vi "Kaelus PFE Initialize.vi"(8 "error in (no error)":errorcluster, 11 "Configuration":T2={"BusType"=enum."USB", "Card"=0, "USB"="", "IP"=0, "COM"=1, "Baud Rate"=enum."9600"}) -> (0 "error out":errorcluster {"code" format="%.0x"}, 3 "DAQmx Dev Name (FEModule)":string, 5 "Kaelus PFE":T1)   [LabVIEW 2011]
uses:
  TypeDefs/Kaelus PFE Configuration.ctl
  TypeDefs/Kaelus PFE Instrument Info.ctl
  OpenG.LIB/file/file.llb/File Exists - Scalar__ogtk.vi
  <vilib>/Utility/config.llb/Read Key (String).vi
  <vilib>/Utility/config.llb/NI_LVConfig.lvlib
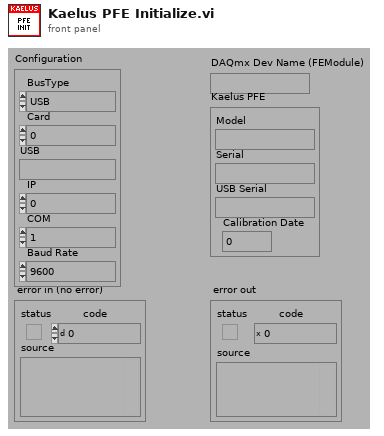
[diagram p1: front panel]
types:
  T1 = typedef "Kaelus PFE Instrument Info.ctl" = cluster{"Model":string, "Serial":string, "USB Serial":string, "Calibration Date":dbl}
  T2 = typedef "Kaelus PFE Configuration.ctl" = cluster{"BusType":enum32{"PCI/ISA/PCMCIA", "USB", "Ethernet", "Serial"}, "Card":i32, "USB":string, "IP":u32, "COM":i32, "Baud Rate":enum16{"300", "600", "1200", "2400", "4800", "9600"}}
  T3 = enum32{"invalid app kind", "Development System", "Run Time System", "Student Edition", "Embedded LabVIEW", "Evaluation", "Custom"}
  T4 = enum32{"PCI/ISA/PCMCIA", "USB", "Ethernet", "Serial"}
  T5 = enum16{"300", "600", "1200", "2400", "4800", "9600"}
  T6 = typedef "ModuleDef.ctl" = cluster{"DevName":string, "DevDetails":string, "DevID":u32, "HW Present":bool, "Module ID":u16, "ModuleCAL":path, "Module Type":T7, "Valid Cal?":bool, "UID":string}
  T7 = typedef "Module_Types.ctl" = enum16{"Unknown", "RF Module", "PA Module", "TR Module", "FE Module", "SW Module"}
  T8 = typedef "NI_LVConfig.lvlib/Config Data RefNum.ctl" = refnum<k1>
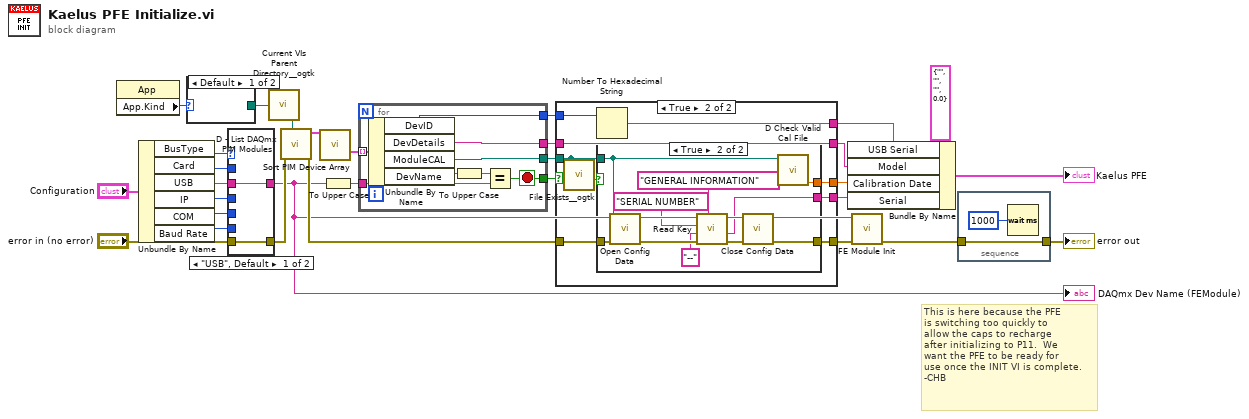
[diagram p0: block diagram]
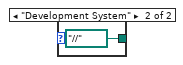
[diagram p2: hidden frame]
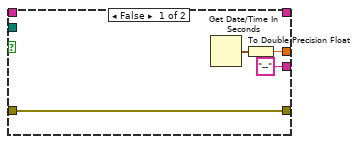
[diagram p3: hidden frame]
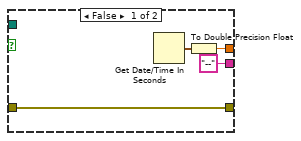
[diagram p4: hidden frame]
diagram:
  # "This is here because the PFE\nis switching too quickly to\nallow the caps to recharge\nafter initializing to P11.  We\nwant the PFE to be ready for\nuse once the INIT VI is complete.\n-CHB"
  n1 = property class="App"() -> ("App.Kind"=w10:T3)  [unwired: 2 in, 2 out]
  n2 = Unbundle By Name("Configuration") -> ("BusType"=w29:T4, "Card"=w28:i32, "USB"=w27:string, "IP"=w26:u32, "COM"=w25:i32, "Baud Rate"=w23:T5)
  n3 = case shown="Default" w10 {
    tunnel: [_ path "../../.." ("Relative path (.)")] -> w9
    frame Default {
    }
    frame "Development System" {
    }
  }
  n4 = case shown="\"USB\", Default" w29 {
    tunnel: "error in (no error)" -> [w33 w34]
    tunnel: w28 -> [_ _]
    tunnel: w27 -> [w32 _]
    tunnel: w26 -> [_ _]
    tunnel: w25 -> [_ _]
    tunnel: [w33 w34] -> w19
    tunnel: [w32 _] -> w11
    tunnel: w23 -> [_ _]
    frame "USB", Default {
    }
    frame "PCI/ISA/PCMCIA", "Ethernet", "Serial" {
    }
  }
  "DAQmx Dev Name (FEModule)" <- w11
  n5 = call "Current VIs Parent Directory__ogtk.vi"("Relative path (.)"=w9) -> ("Parent Directory (+ Relative)"=w8:path)  [unwired: 4 in]
  n6 = call "D - List DAQmx PIM Modules.vi"("Cal Folder Path"=w8, "error in (no error)"=w19) -> ("error out"=w15:errorcluster, "PIM Modules"=w17:T6[])  [unwired: 8 in]
  n7 = call "Sort PIM Device Array.vi"("PIM Devices"=w17) -> ("FE Devices"=w6:T6[])  [unwired: 8 in, 6 out]
  n8 = To Upper Case(1:w11) -> (0:w16:string)
  n9 = for {
    tunnel: w16 -> [w41]
    tunnel: [w39] -> w14
    tunnel: [w38] -> w12
    tunnel: [w37] -> w13
    tunnel: w6 -> [w36] mode=indexing
    tunnel: [w35] -> w5
    stop <- w37 stop-if-true
    n10 = Unbundle By Name(w36) -> ("DevID"=w35:u32, "DevDetails"=w38:string, "ModuleCAL"=w39:path, "DevName"=w42:string)
    n11 = To Upper Case(1:w42) -> (0:w40:string)
    n12 = Equal?(x=w40, y=w41) -> (x = y?=w37:bool)
  }
  n13 = case shown="True" w13 {
    tunnel: w15 -> [w46 w55]
    tunnel: [w46 w54] -> w18
    tunnel: w14 -> [_ w53]
    tunnel: ["--" ("value") w51] -> w21
    tunnel: [w43 w50] -> w7
    tunnel: w12 -> [_ w49]
    tunnel: [_ w49] -> w4
    tunnel: w5 -> [_ w48]
    tunnel: [_ w47] -> w3
    frame False {
      n14 = Get Date/Time In Seconds() -> (seconds since 1Jan1904=w44:timestamp)
      n15 = To Double Precision Float(number=w44) -> (double precision float=w43:dbl)
    }
    frame True {
      n16 = call-poly "File Exists__ogtk.vi"("file path"=w53) -> ("exists"=w52:bool)  [unwired: 6 in, 1 out]
      n17 = Number To Hexadecimal String(2:w48) -> (0:w47:string)  [unwired: 1 in]
      n18 = case shown="True" w52 {
        tunnel: w55 -> [w59 w67]
        tunnel: [w59 w64] -> w54
        tunnel: w53 -> [_ w61]
        tunnel: ["--" ("value") w63] -> w51
        tunnel: [w56 w60] -> w50
        frame False {
          n19 = Get Date/Time In Seconds() -> (seconds since 1Jan1904=w57:timestamp)
          n20 = To Double Precision Float(number=w57) -> (double precision float=w56:dbl)
        }
        frame True {
          n21 = call <vilib>:"Open Config Data.vi"("error in (no error)"=w67, "configuration file path"=w61) -> ("error out"=w69:errorcluster, "refnum"=w65:T8)  [unwired: 7 in, 1 out]
          n22 = call-poly <vilib>:"Read Key.vi"("section"="GENERAL INFORMATION", "error in (no error)"=w69, "default value"="--", "key"="SERIAL NUMBER", "refnum"=w65) -> ("error out"=w68:errorcluster, "value"=w63:string, "refnum out"=w66:T8)  [unwired: 1 in, 3 out]
          n23 = call <vilib>:"Close Config Data.vi"("error in (no error)"=w68, "refnum"=w66) -> ("error out"=w64:errorcluster)  [unwired: 8 in, 1 out]
          n24 = call "D Check Valid Cal File.vi"("Device Cal File Path"=w61) -> ("Cal Date"=w60:dbl)  [unwired: 10 out]
        }
      }
    }
  }
  n25 = Bundle By Name(cluster=T1 {"Model"="", "Serial"="", "USB Serial"="", "Calibration Date"=0.0} ("Kaelus SWI"), "USB Serial"=w3, "Model"=w4, "Calibration Date"=w7, "Serial"=w21) -> (→"Kaelus PFE":T1)
  n26 = call "FE Module Init.vi"("error in (no error)"=w18, "DAQmx Dev Name (PIM_FEModule)"=w11) -> ("error out"=w2:errorcluster)  [unwired: 3 in, 2 out]
  n27 = stacked-sequence {
    tunnel: w2 -> [w72]
    tunnel: [w72] -> w1
    frame #0 {
      n28 = Wait (ms)(milliseconds to wait=u32 1000) -> ()  [unwired: 1 out]
    }
  }
  "error out" <- w1
